vi "Parking Go.vi"(8 "error in (no error)":errorcluster, 11 "A3200 in":refnum<class "A3200.lvclass">) -> (0 "error out":errorcluster, 3 "A3200 out":refnum<class "A3200.lvclass">)   [LabVIEW 2016]
uses:
  A3200.lvclass
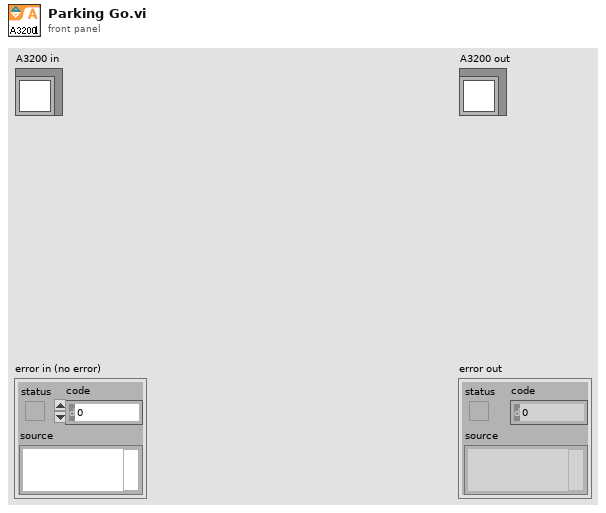
[diagram p1: front panel]
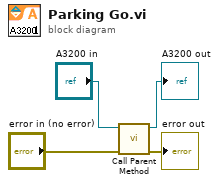
[diagram p0: block diagram]
diagram:
  n1 = call-parent "Call Parent Method"("error in (no error)"="error in (no error)", "Motion in"="A3200 in") -> ("error out"=→"error out":errorcluster, "Motion out"=→"A3200 out":refnum<class "A3200.lvclass">)  [unwired: 8 in]
